vi "RT Loop - Config Calibration.vi"(11 "Message Queue":refnum<queue>) -> ()   [LabVIEW 2018]
doc: "This RSI Control Loop VI performs control calculations on four input channels in parallel, and outputs the results to four output channels."
uses:
  Support/Message Queue/Message Cluster.ctl
  Support/Message Queue/Message.ctl
  <vilib>/Platform/TimedLoop/XDataNode/timing_clust.ctl
  <vilib>/Platform/TimedLoop/XDataNode/nitl_modes.ctl
  <vilib>/Platform/TimedLoop/XDataNode/wakeup.ctl
  Controls/ConfigCalibration.ctl
  <vilib>/Platform/TimedLoop/XDataNode/loadnilvce.vi
  <vilib>/Platform/TimedLoop/XDataNode/XDataNode.xnode
  <vilib>/Platform/TimedLoop/XDataNode/XDNodeRunTimeDep.lvlib
  support/Message Queue/Message Queue.lvlib
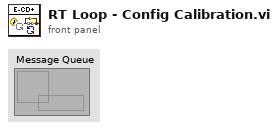
[diagram p1: front panel]
types:
  T1 = typedef "XDNodeRunTimeDep.lvlib/timing_clust.ctl" = cluster{"Expected End [f-1]":u64, "Actual End [f-1]":u64, "Finished Late? [f-1]":bool, "Expected End [i-1]":u64, "Actual End [i-1]":u64, "Finished Late? [i-1]":bool, "Expected Start [i]":u64, "Actual Start [i]":u64, "Expected Start [f]":u64, "Actual Start [f]":u64, "Source Name":string, "Structure Name":string, "Period":i64, "Deadline":i64, "Offset":i64, "Start":i64, "Priority":i32, "Timeout":i32, "Mode":T2, "Wakeup Reason":T3, "Error":errorcluster, "Source Type":string, "Secondary Source Type":string, "Global End Time":u64, "Global Start Time":u64, "Frame Duration":u64, "Iteration Duration":u64, "Assigned CPU":i32, "I/O Scan Engine Mode":u32}
  T2 = typedef "XDNodeRunTimeDep.lvlib/nitl_modes.ctl" = enum32{"No Change", "Process missed periods, maintain original phase", "Discard missed periods, maintain original phase", "Process missed periods, ignore original phase", "Discard missed periods, ignore original phase"}
  T3 = typedef "XDNodeRunTimeDep.lvlib/wakeup.ctl" = enum32{"Normal", "Aborted", "Asynchronous wakeup", "Timing source error", "Timed loop error", "Timeout"}
  T4 = typedef "ConfigCalibration.ctl" = enum16{"CAL STOP", "TWTT OP (IN)", "TWTT PDP (IN)", "DLT OP (IN)", "DLT PDP 01 (IN)", "DLT PDP 02 (IN)", "BR OP (IN)", "BR TWT ALIGN (IN)", "BR DL ALIGN (IN)"}
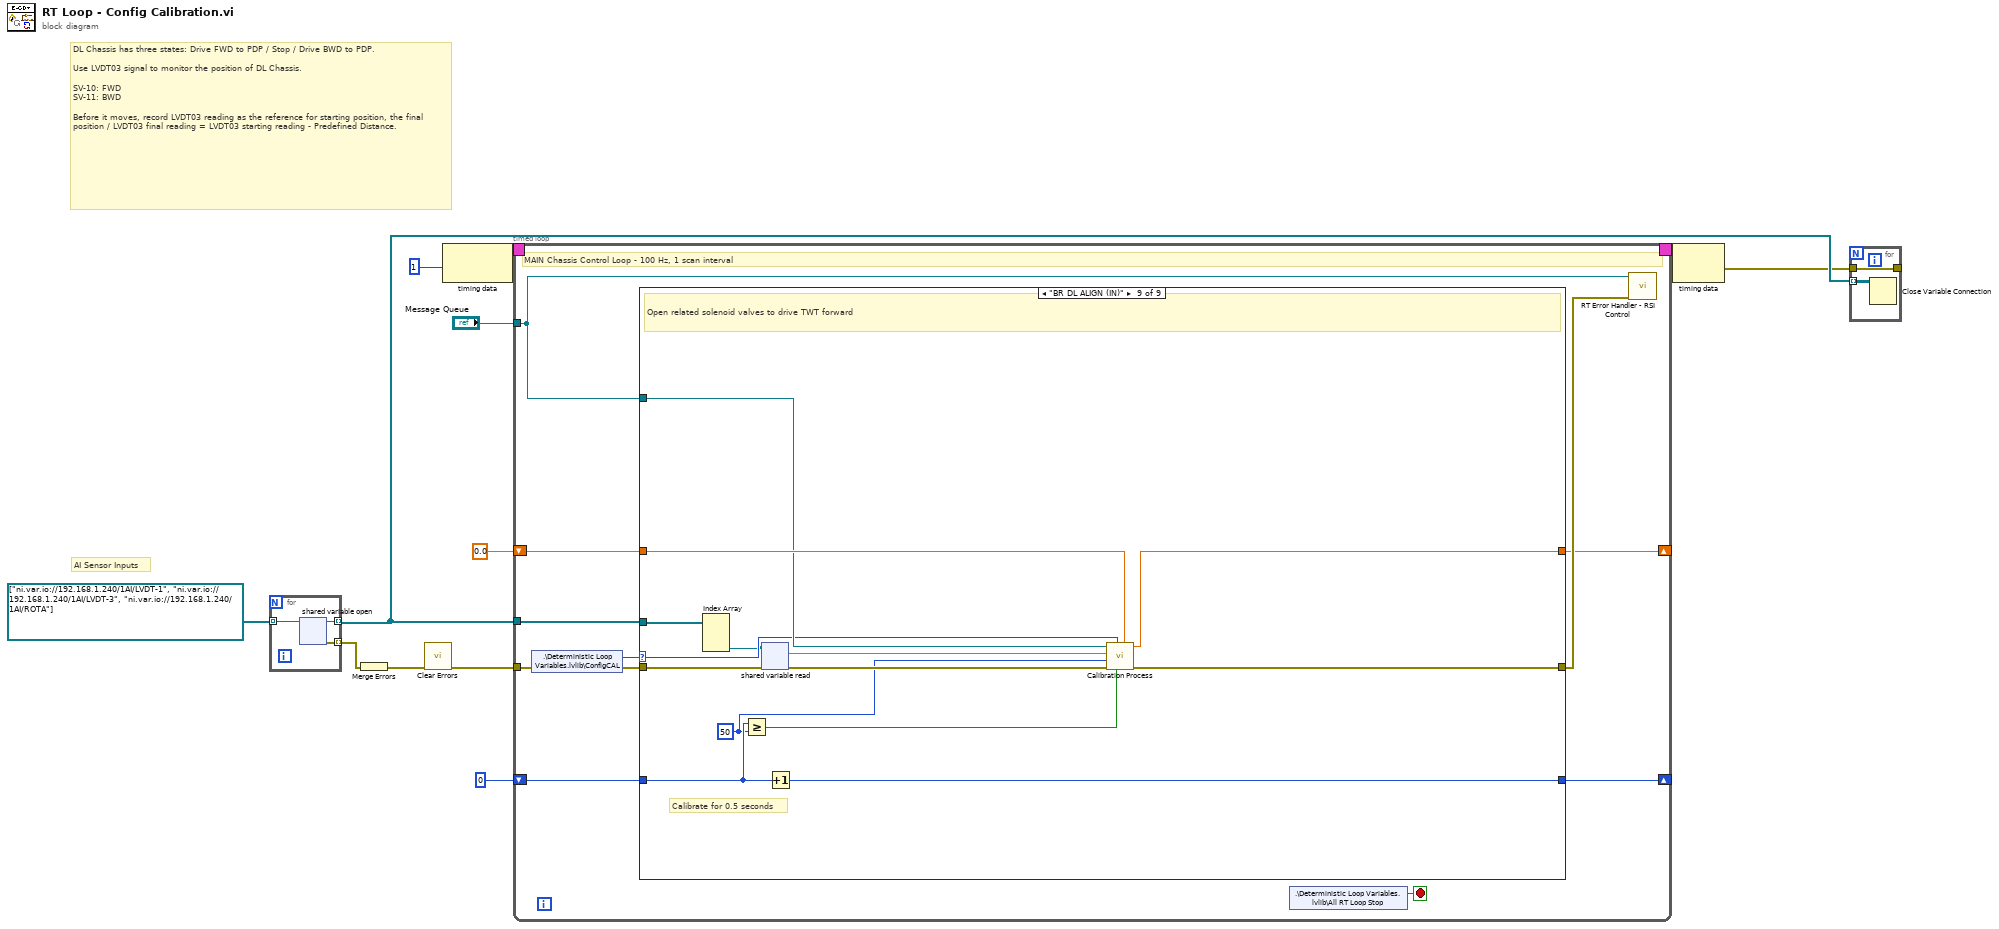
[diagram p0: block diagram]
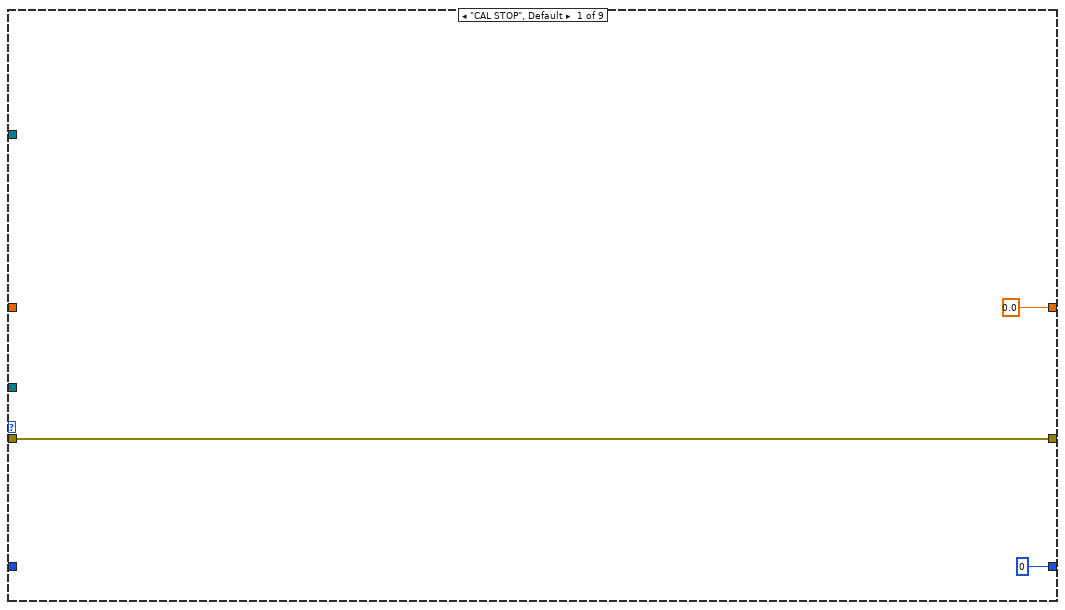
[diagram p2: hidden frame]
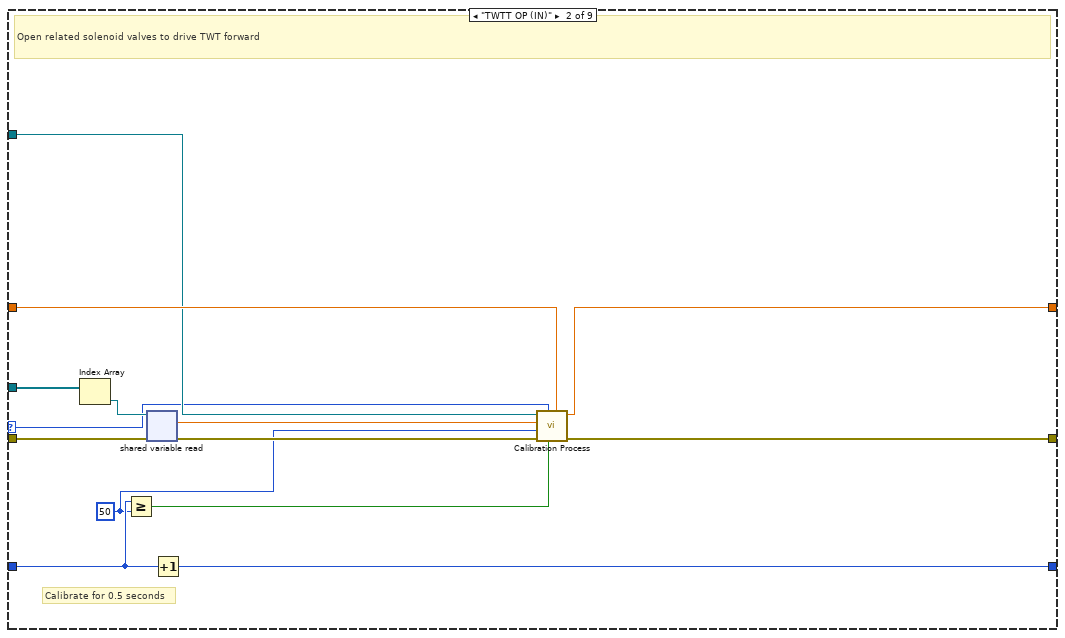
[diagram p3: hidden frame]
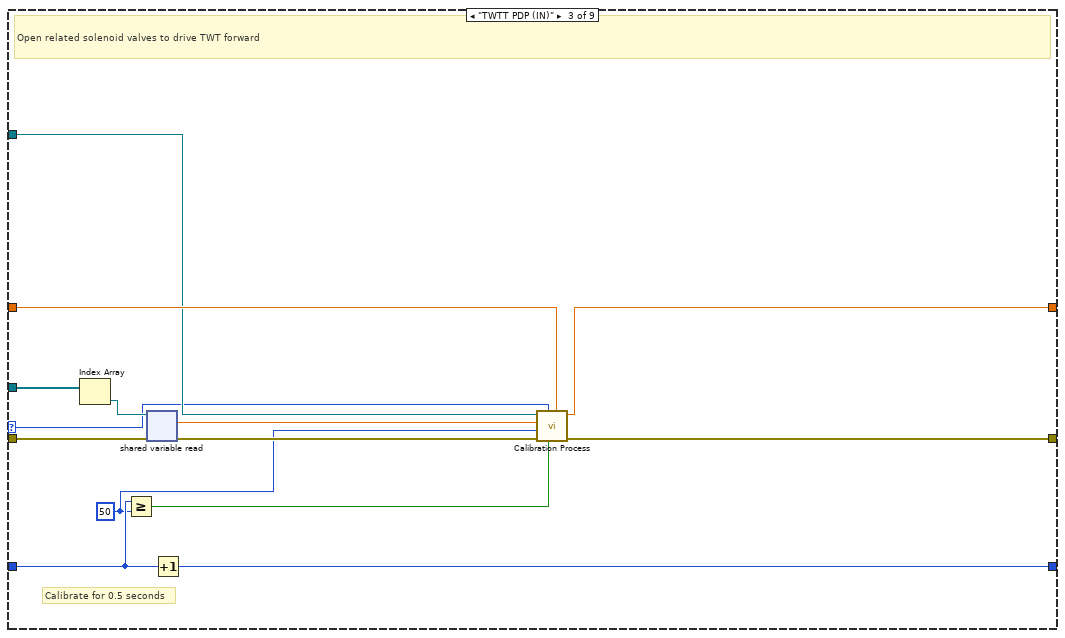
[diagram p4: hidden frame]
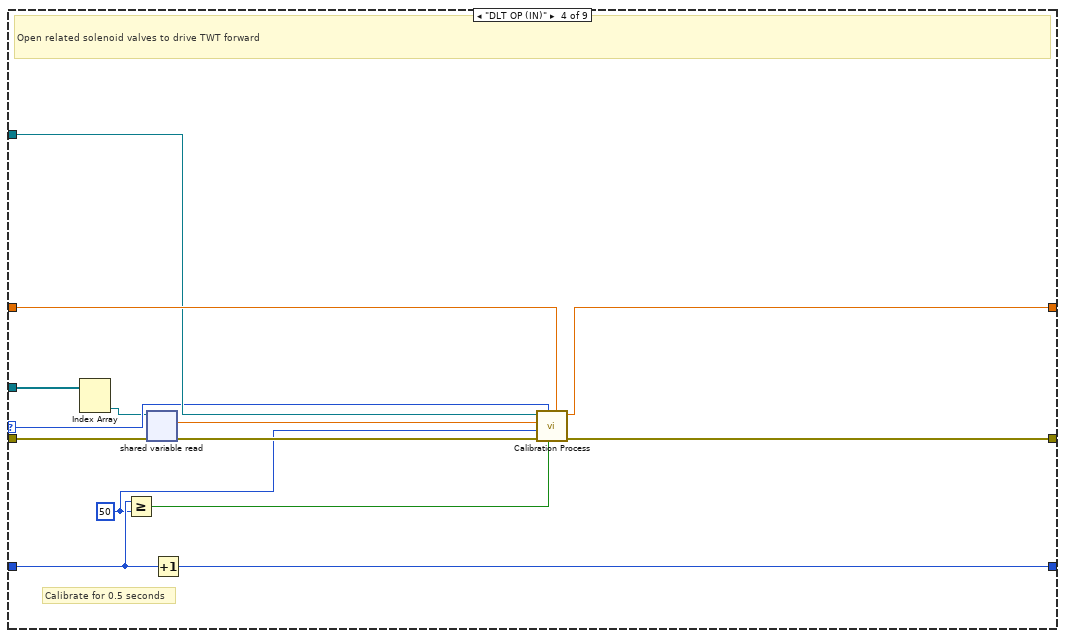
[diagram p5: hidden frame]
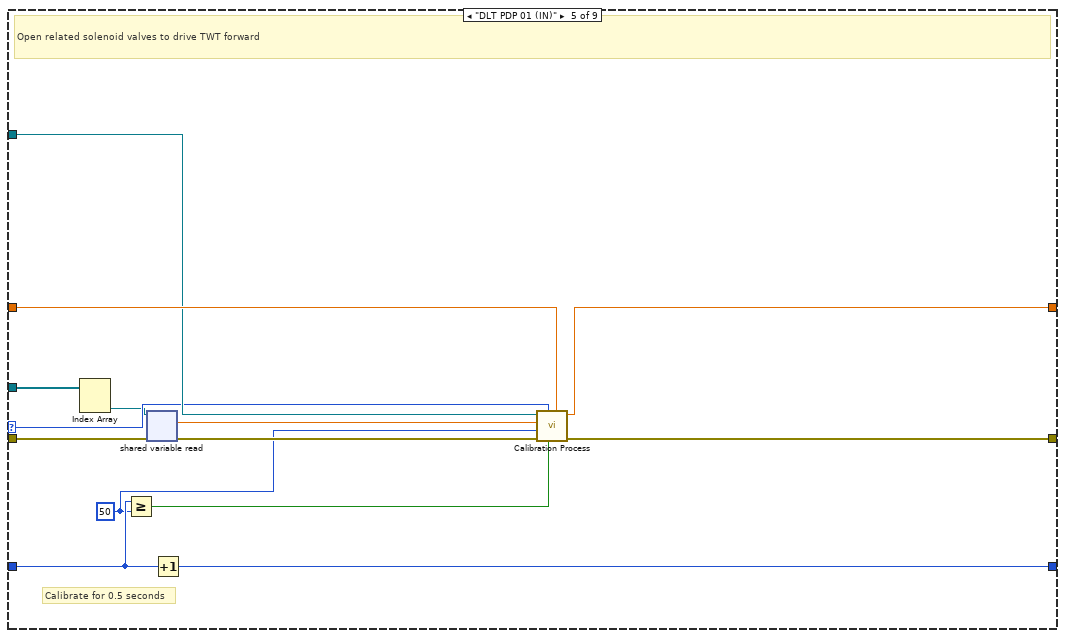
[diagram p6: hidden frame]
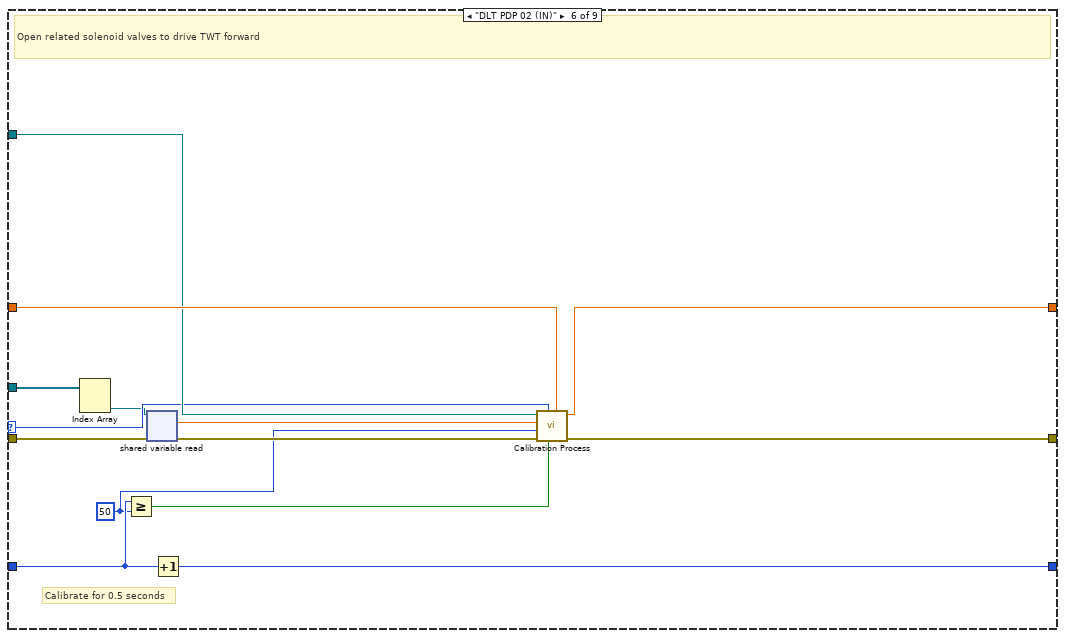
[diagram p7: hidden frame]
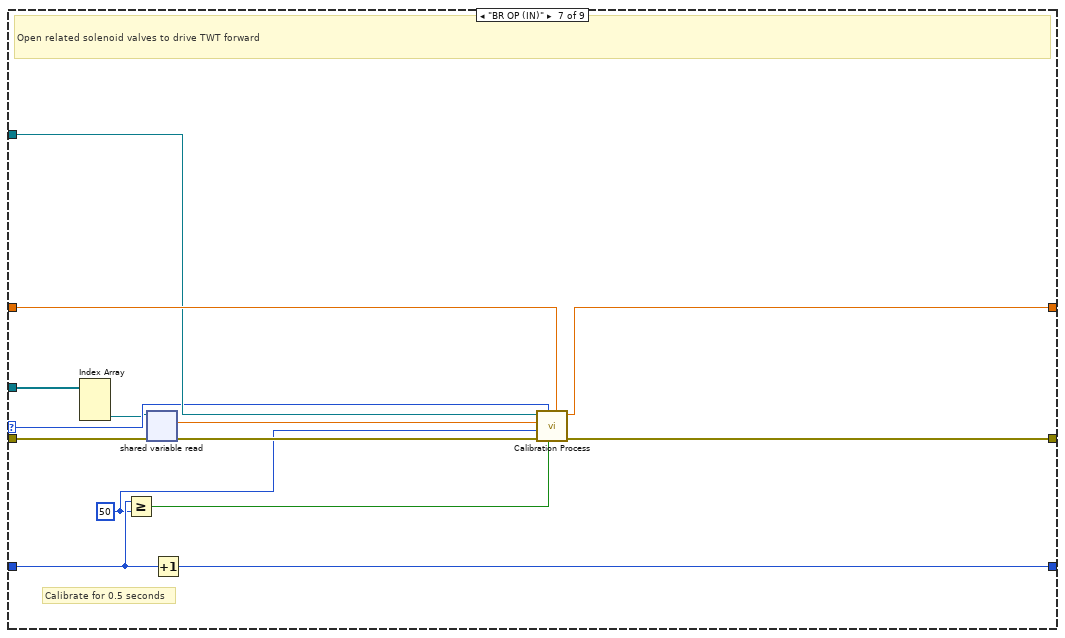
[diagram p8: hidden frame]
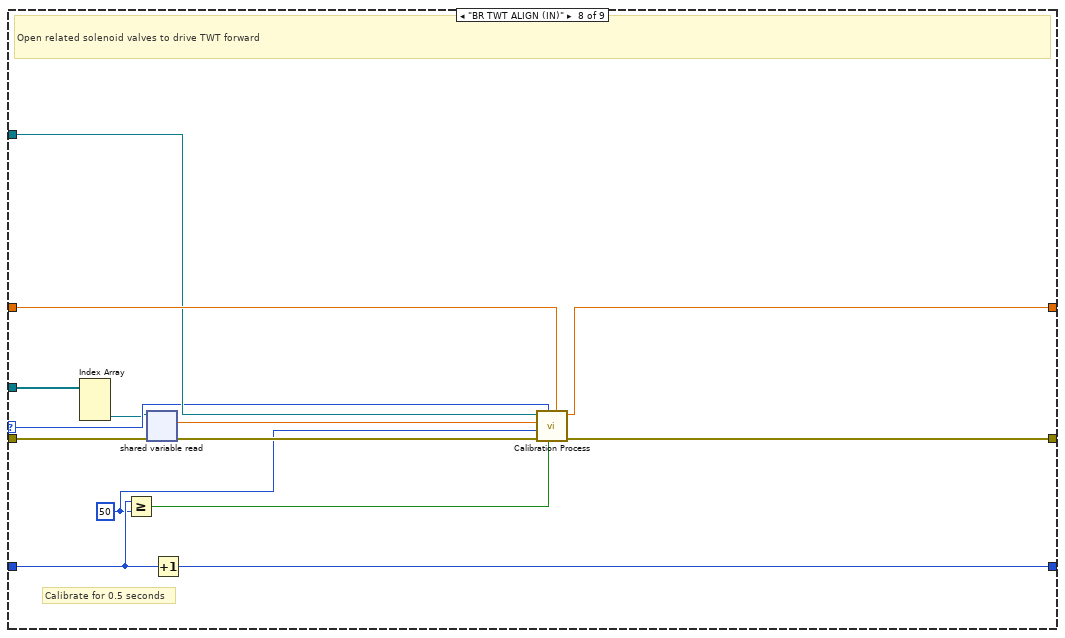
[diagram p9: hidden frame]
diagram:
  # "AI Sensor Inputs"
  # "DL Chassis has three states: Drive FWD to PDP / Stop / Drive BWD to PDP.\n\nUse LVDT03 signal to monitor the position of DL Chassis.\n\nSV-10: FWD\nSV-11: BWD\n\nBefore it moves, record LVDT03 reading as the reference for starting position, the final position / LVDT03 final reading = LVDT03 starting reading - Predefined Distance."
  n1 = for {
    tunnel: refnum<k21>[] ["ni.var.io://192.168.1.240/1AI/LVDT-1", "ni.var.io://192.168.1.240/1AI/LVDT-3", "ni.var.io://192.168.1.240/1AI/ROTA"] -> [w15] mode=indexing
    tunnel: [w13] -> w6 mode=indexing
    tunnel: [w14] -> w3 mode=indexing
    n2 = shared-variable-open(w15) -> (w13:refnum<k21>, w14:errorcluster)  [unwired: 1 in]
  }
  n3 = Merge Errors(w3) -> (w4:errorcluster)
  n4 = call <vilib>:"Clear Errors.vi"("error in (no error)"=w4) -> ("error out"=w7:errorcluster)  [unwired: 5 in, 1 out]
  n5 = node-c288(i64 1 ("Period")) -> (w12:T1)
  n6 = timed-loop "Timed Loop" {
    timing: w12 -> [_]
    timing-out: [_] -> w11
    tunnel: "Message Queue" -> [w20]
    tunnel: w7 -> [w23]
    tunnel: w6 -> [w25]
    shift-right: [w18] -> _
    shift-left: 0.0 -> [w19]
    shift-right: [w16] -> _
    shift-left: 0 -> [w17]
    stop <- w26 stop-if-true
    # "MAIN Chassis Control Loop - 100 Hz, 1 scan interval"
    n7 = shared-variable ".\\Deterministic Loop Variables.lvlib\\ConfigCAL"(error in=w23) -> (w24:T4, error out=w22:errorcluster)
    n8 = case shown="\"BR DL ALIGN (IN)\"" w24 {
      selector: w24 -> [_ w31 w45 w60 w74 w88 w102 w116 w130]
      tunnel: w25 -> [_ w43 w57 w71 w85 w99 w113 w127 w141]
      tunnel: w22 -> [w29 w41 w55 w70 w84 w98 w112 w126 w140]
      tunnel: [w29 w35 w49 w64 w78 w92 w106 w120 w134] -> w21
      tunnel: w20 -> [_ w32 w46 w61 w75 w89 w103 w117 w131]
      tunnel: w19 -> [_ w39 w53 w68 w82 w96 w110 w124 w138]
      tunnel: [0.0 w34 w48 w63 w77 w91 w105 w119 w133] -> w18
      tunnel: w17 -> [_ w38 w52 w67 w81 w95 w109 w123 w137]
      tunnel: [0 w37 w51 w66 w80 w94 w108 w122 w136] -> w16
      frame "CAL STOP", Default {
      }
      frame "TWTT OP (IN)" {
        w33 = 50 ("y")
        # "Calibrate for 0.5 seconds"
        # "Open related solenoid valves to drive TWT forward"
        n9 = Index Array(array=w43) -> (element=w42:refnum<k21>)  [unwired: 1 in]
        n10 = Greater Or Equal?(x=w38, y=w33) -> (x >= y?=w40:bool)
        n11 = shared-variable-read(w42, w41) -> (w36:errorcluster, w30:dbl)  [unwired: 1 out]
        n12 = Increment(x=w38) -> (x+1=w37:i32)
        n13 = call "Calibration Process.vi"("Sum in"=w39, "DONE?"=w40, "CONFIG CALIBRATION"=w31, "error in"=w36, "Index"=w33, "Current Valve"=w30, "Queue in"=w32) -> ("error out"=w35:errorcluster, "Sum out"=w34:dbl)  [unwired: 3 in]
      }
      frame "TWTT PDP (IN)" {
        w47 = 50 ("y")
        # "Calibrate for 0.5 seconds"
        # "Open related solenoid valves to drive TWT forward"
        n14 = Index Array(array=w57) -> (element=w56:refnum<k21>)  [unwired: 1 in]
        n15 = Greater Or Equal?(x=w52, y=w47) -> (x >= y?=w54:bool)
        n16 = shared-variable-read(w56, w55) -> (w50:errorcluster, w44:dbl)  [unwired: 1 out]
        n17 = Increment(x=w52) -> (x+1=w51:i32)
        n18 = call "Calibration Process.vi"("Sum in"=w53, "DONE?"=w54, "CONFIG CALIBRATION"=w45, "error in"=w50, "Index"=w47, "Current Valve"=w44, "Queue in"=w46) -> ("error out"=w49:errorcluster, "Sum out"=w48:dbl)  [unwired: 3 in]
      }
      frame "DLT OP (IN)" {
        w62 = 50 ("y")
        # "Calibrate for 0.5 seconds"
        # "Open related solenoid valves to drive TWT forward"
        n19 = Index Array(array=w71) -> (element #2=w58:refnum<k21>)  [unwired: 2 in, 1 out]
        n20 = Greater Or Equal?(x=w67, y=w62) -> (x >= y?=w69:bool)
        n21 = shared-variable-read(w58, w70) -> (w65:errorcluster, w59:dbl)  [unwired: 1 out]
        n22 = Increment(x=w67) -> (x+1=w66:i32)
        n23 = call "Calibration Process.vi"("Sum in"=w68, "DONE?"=w69, "CONFIG CALIBRATION"=w60, "error in"=w65, "Index"=w62, "Current Valve"=w59, "Queue in"=w61) -> ("error out"=w64:errorcluster, "Sum out"=w63:dbl)  [unwired: 3 in]
      }
      frame "DLT PDP 01 (IN)" {
        w76 = 50 ("y")
        # "Calibrate for 0.5 seconds"
        # "Open related solenoid valves to drive TWT forward"
        n24 = Index Array(array=w85) -> (element #2=w72:refnum<k21>)  [unwired: 2 in, 1 out]
        n25 = Greater Or Equal?(x=w81, y=w76) -> (x >= y?=w83:bool)
        n26 = shared-variable-read(w72, w84) -> (w79:errorcluster, w73:dbl)  [unwired: 1 out]
        n27 = Increment(x=w81) -> (x+1=w80:i32)
        n28 = call "Calibration Process.vi"("Sum in"=w82, "DONE?"=w83, "CONFIG CALIBRATION"=w74, "error in"=w79, "Index"=w76, "Current Valve"=w73, "Queue in"=w75) -> ("error out"=w78:errorcluster, "Sum out"=w77:dbl)  [unwired: 3 in]
      }
      frame "DLT PDP 02 (IN)" {
        w90 = 50 ("y")
        # "Calibrate for 0.5 seconds"
        # "Open related solenoid valves to drive TWT forward"
        n29 = Index Array(array=w99) -> (element #2=w86:refnum<k21>)  [unwired: 2 in, 1 out]
        n30 = Greater Or Equal?(x=w95, y=w90) -> (x >= y?=w97:bool)
        n31 = shared-variable-read(w86, w98) -> (w93:errorcluster, w87:dbl)  [unwired: 1 out]
        n32 = Increment(x=w95) -> (x+1=w94:i32)
        n33 = call "Calibration Process.vi"("Sum in"=w96, "DONE?"=w97, "CONFIG CALIBRATION"=w88, "error in"=w93, "Index"=w90, "Current Valve"=w87, "Queue in"=w89) -> ("error out"=w92:errorcluster, "Sum out"=w91:dbl)  [unwired: 3 in]
      }
      frame "BR OP (IN)" {
        w104 = 50 ("y")
        # "Calibrate for 0.5 seconds"
        # "Open related solenoid valves to drive TWT forward"
        n34 = Index Array(array=w113) -> (element #3=w100:refnum<k21>)  [unwired: 3 in, 2 out]
        n35 = Greater Or Equal?(x=w109, y=w104) -> (x >= y?=w111:bool)
        n36 = shared-variable-read(w100, w112) -> (w107:errorcluster, w101:dbl)  [unwired: 1 out]
        n37 = Increment(x=w109) -> (x+1=w108:i32)
        n38 = call "Calibration Process.vi"("Sum in"=w110, "DONE?"=w111, "CONFIG CALIBRATION"=w102, "error in"=w107, "Index"=w104, "Current Valve"=w101, "Queue in"=w103) -> ("error out"=w106:errorcluster, "Sum out"=w105:dbl)  [unwired: 3 in]
      }
      frame "BR TWT ALIGN (IN)" {
        w118 = 50 ("y")
        # "Calibrate for 0.5 seconds"
        # "Open related solenoid valves to drive TWT forward"
        n39 = Index Array(array=w127) -> (element #3=w114:refnum<k21>)  [unwired: 3 in, 2 out]
        n40 = Greater Or Equal?(x=w123, y=w118) -> (x >= y?=w125:bool)
        n41 = shared-variable-read(w114, w126) -> (w121:errorcluster, w115:dbl)  [unwired: 1 out]
        n42 = Increment(x=w123) -> (x+1=w122:i32)
        n43 = call "Calibration Process.vi"("Sum in"=w124, "DONE?"=w125, "CONFIG CALIBRATION"=w116, "error in"=w121, "Index"=w118, "Current Valve"=w115, "Queue in"=w117) -> ("error out"=w120:errorcluster, "Sum out"=w119:dbl)  [unwired: 3 in]
      }
      frame "BR DL ALIGN (IN)" {
        w132 = 50 ("y")
        # "Calibrate for 0.5 seconds"
        # "Open related solenoid valves to drive TWT forward"
        n44 = Index Array(array=w141) -> (element #3=w128:refnum<k21>)  [unwired: 3 in, 2 out]
        n45 = Greater Or Equal?(x=w137, y=w132) -> (x >= y?=w139:bool)
        n46 = shared-variable-read(w128, w140) -> (w135:errorcluster, w129:dbl)  [unwired: 1 out]
        n47 = Increment(x=w137) -> (x+1=w136:i32)
        n48 = call "Calibration Process.vi"("Sum in"=w138, "DONE?"=w139, "CONFIG CALIBRATION"=w130, "error in"=w135, "Index"=w132, "Current Valve"=w129, "Queue in"=w131) -> ("error out"=w134:errorcluster, "Sum out"=w133:dbl)  [unwired: 3 in]
      }
    }
    n49 = shared-variable ".\\Deterministic Loop Variables.lvlib\\All RT Loop Stop"() -> (w26:bool)  [unwired: 1 in, 1 out]
    n50 = call "RT Error Handler - RSI Control.vi"("error in (no error)"=w21, "Message Queue"=w20) -> ()  [unwired: 8 in, 2 out]
  }
  n51 = node-c288(w11) -> (w5:errorcluster)
  n52 = for {
    tunnel: w5 -> [w144]
    tunnel: w6 -> [w145] mode=indexing
    tunnel: [w144] -> _
    n53 = Close Variable Connection(11:w145) -> ()  [unwired: 1 in, 1 out]
  }
